vi "var_string.vi"() -> ()   [LabVIEW 2009]
panel:
  out "Afisare text":string
  in  "Introduceti un text":string
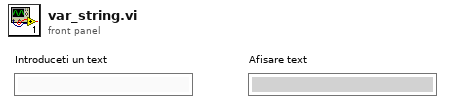
[diagram p1: front panel]
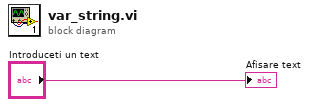
[diagram p0: block diagram]
diagram:
  "Afisare text" <- "Introduceti un text"
